vi "Joystick1_YAxis.vi"() -> ()   [LabVIEW 2016]
panel:
  out "Joystick1_YAxis":dbl
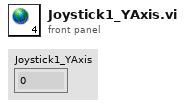
[diagram p1: front panel]
diagram:
